vi "EMV T6 T7 Flow Detect.vi"(0 "T7 Detect?":bool, 1 "Current T6 Temperatures":dbl[](array[numeric]), 2 "Absolute Delta T6":dbl, 5 "T6_OFFSET_FROM_TARGET_INDICATING_FLOW":dbl=3.0, 7 "T6_DELTA_INDICATING_FLOW":dbl=2.0, 11 "error in (no error)":errorcluster, 12 "User Setpoint Temperature":u16=125) -> (4 "Flow Dectection":bool, 15 "error out":errorcluster)   [LabVIEW 2016]
panel:
  # "T6 Data"
  # "Basic Inputs"
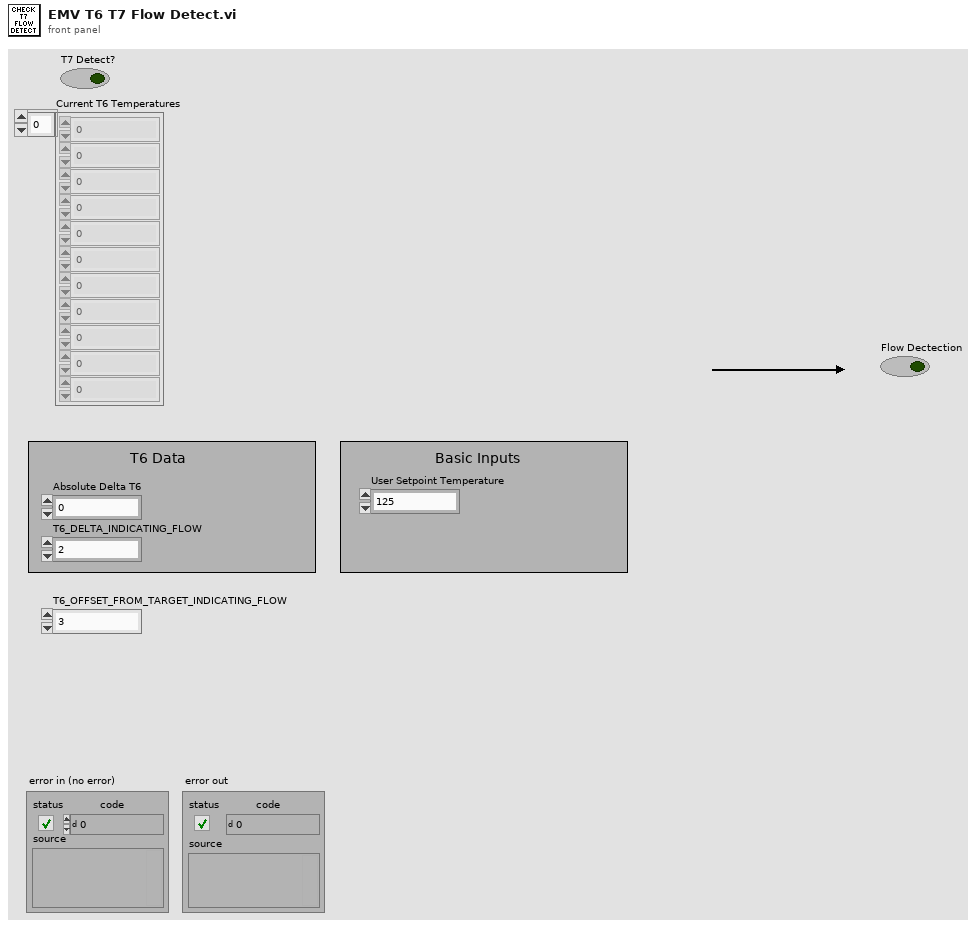
[diagram p1: front panel]
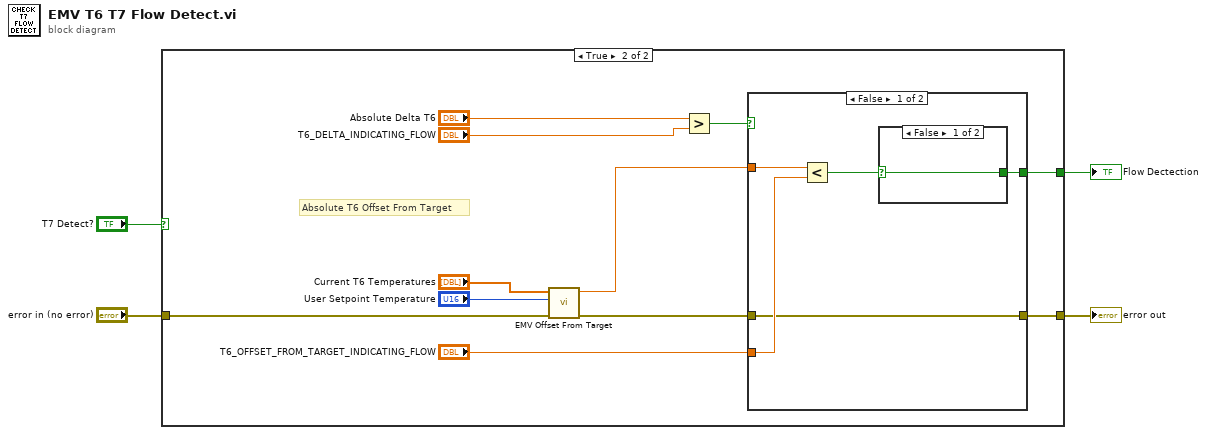
[diagram p0: block diagram]
diagram:
  n1 = case shown="True" "T7 Detect?" {
    selector: "T7 Detect?" -> [w6 _]
    tunnel: [w6 w16] -> w4
    tunnel: "error in (no error)" -> [w5 w9]
    tunnel: [w5 w7] -> w1
    frame False {
    }
    frame True {
      # "Absolute T6 Offset From Target"
      n2 = call "EMV Offset From Target.vi"("error in (no error)"=w9, "User Setpoint Temperature"="User Setpoint Temperature", "Current T6 Temperatures"="Current T6 Temperatures") -> ("error out"=w8:errorcluster, "Absolute T6 Offset From Target"=w10:dbl)  [unwired: 7 in]
      n3 = Greater?(x="Absolute Delta T6", y="T6_DELTA_INDICATING_FLOW") -> (0:w17:bool)
      n4 = case shown="False" w17 {
        selector: w17 -> [_ w26]
        tunnel: [w20 w26] -> w16
        tunnel: w10 -> [w22 _]
        tunnel: "T6_OFFSET_FROM_TARGET_INDICATING_FLOW" -> [w19 _]
        tunnel: [w18 w25] -> w7
        tunnel: w8 -> [w18 w25]
        frame False {
          n5 = Less?(x=w22, y=w19) -> (x < y?=w21:bool)
          n6 = case shown="False" w21 {
            selector: w21 -> [w23 w24]
            tunnel: [w23 w24] -> w20
            frame False {
            }
            frame True {
            }
          }
        }
        frame True {
          # "There is a constant\nthat helps determine \nflow assuming a T6/T7 \ndetect"
        }
      }
    }
  }
  "Flow Dectection" <- w4
  "error out" <- w1
